vi "Check UID Empty.vi"(10 "UID":string) -> (2 "Error":errorcluster)   [LabVIEW 2020, in "jettl.lvlib"]
uses:
  jettl.lvlib
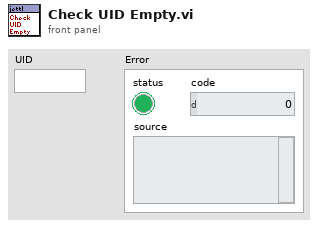
[diagram p1: front panel]
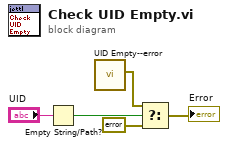
[diagram p0: block diagram]
diagram:
  n1 = Empty String/Path?(string/path="UID") -> (empty?=w3:bool)
  n2 = call "UID Empty--error.vi"() -> ("Error"=w4:errorcluster)  [unwired: 11 in]
  n3 = Select(t=w4, s=w3, f=errorcluster {"status"=FALSE, "code"=0, "source"=""}) -> (s? t:f=→"Error":errorcluster)
